vi "calibration function CO2.vi"(7 "x":dbl) -> (8 "f(x)":dbl)   [LabVIEW 2017, in "LicorLI7000.lvlib"]
uses:
  LicorLI7000.lvlib
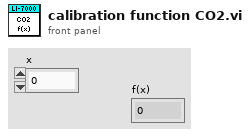
[diagram p1: front panel]
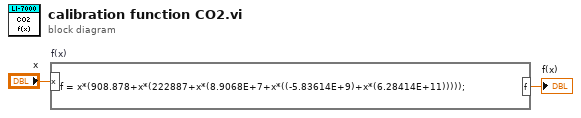
[diagram p0: block diagram]
diagram:
  n1 = formula code="f = x*(908.878+x*(222887+x*(8.9068E+7+x*((-5.83614E+9)+x*(6.28414E+11)))));" "f(x)"("x"="x") -> ("f"=→"f(x)":dbl)
